vi "Execute_remote_call.vi"(0 "Traverse line":T3 {"Row Duration (mins)" format="%#.1f"; "Row No" min=0; "Trace Gas Concentration (%)" min=0.0 format="%#.2f"; "Emission Rate (l/min)" format="%#.2f"; "Tunnel Speed" format="%#.2f"; "Start X" format="%#.2f"; "Start Y" format="%#.2f"; "Start Z" format="%#.2f"; "End X" format="%#.2f"; "End Y" format="%#.2f"; "End Z" format="%#.2f"; "Averaging time (min)" min=0.0 format="%#.2f"}, 2 "Simulate/Run":T2, 3 "VI to run":path) -> (6 "Traverse Out":T3 {"Row Duration (mins)" format="%#.1f"; "Row No" min=0; "Trace Gas Concentration (%)" min=0.0 format="%#.2f"; "Emission Rate (l/min)" format="%#.2f"; "Tunnel Speed" format="%#.2f"; "Start X" format="%#.2f"; "Start Y" format="%#.2f"; "Start Z" format="%#.2f"; "End X" format="%#.2f"; "End Y" format="%#.2f"; "End Z" format="%#.2f"; "Averaging time (min)" min=0.0 format="%#.2f"}, 7 "Status":T1, 8 "Error Messages":string)   [LabVIEW 2012]
uses:
  Traverse_cluster.ctl
  Spacing.ctl
  Controls/Multi_run_mode.ctl
  Controls/User_Specific_mode.ctl
  Multi_Run_Status.ctl
panel:
  # "X           Y            Z"
  # "Start"
  # "End"
  # "X           Y            Z"
  # "Start"
  # "End"
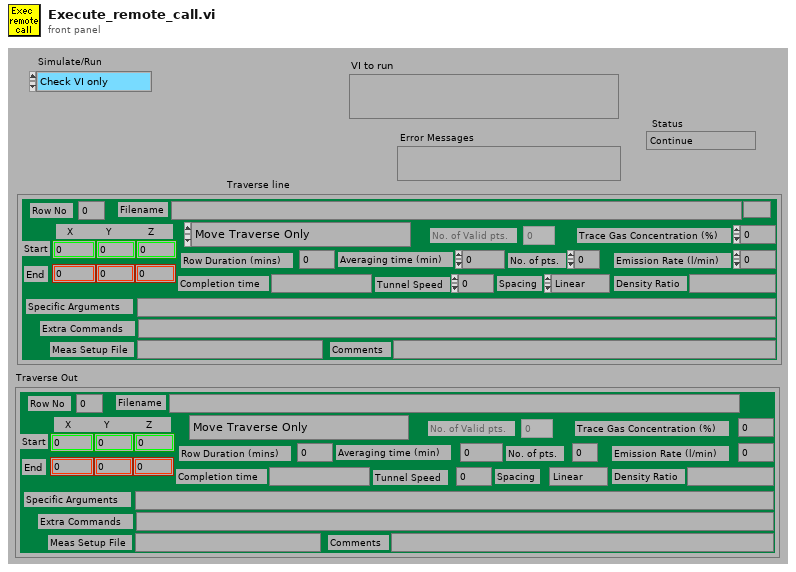
[diagram p1: front panel]
types:
  T1 = typedef "Multi_Run_Status.ctl" = enum16{"Continue", "Jump to Next Point", "Jump to Next Row", "Jump To Fall Back", "Terminate Run"}
  T2 = typedef "User_Specific_mode.ctl" = enum16{"Check VI only", "Run VI"}
  T3 = typedef "Traverse_cluster.ctl" = cluster{"Start X":dbl, "Start Y":dbl, "Start Z":dbl, "End X":dbl, "End Y":dbl, "End Z":dbl, "No. of pts.":i32, "Spacing":T4, "Filename":path, "Tunnel Speed":dbl, "Averaging time (min)":dbl, "Extra Commands":string, "Specific Arguments":string, "Emission Rate (l/min)":dbl, "Trace Gas Concentration (%)":dbl, "Density Ratio":string, "Comments":string, "Row No":i32, "Row Type Selector":T5, "Completion time":string, "Row Duration (mins)":dbl, "No. of Valid pts.":i32, "Meas Setup File":string}
  T4 = typedef "Spacing.ctl" = enum16{"Linear", "Log", "Gauss", "Specified", "N/A"}
  T5 = typedef "Multi_run_mode.ctl" = enum16{"Move Traverse Only", "Set Tunnel Speed Only", "Set Source Only", "Set Measurement Conditions", "Single Measurement", "Vertical Profile", "Lateral Profile", "Longitudinal Profile", "Explore Volume", "Multi-Axis Profile", "Auto Calibrate", "Meas Fast FID Bkgnd", "Check Beam Power", "Scanning Valve Measurement", "Run VI Named:", "Set ADAM Ch", "Wait (minutes)", "Send Message", "Synchronize With:", "Fall Back to this Row", "Turn Off Row Repeating", "Blank Row", "Traverse 3D Volume"}
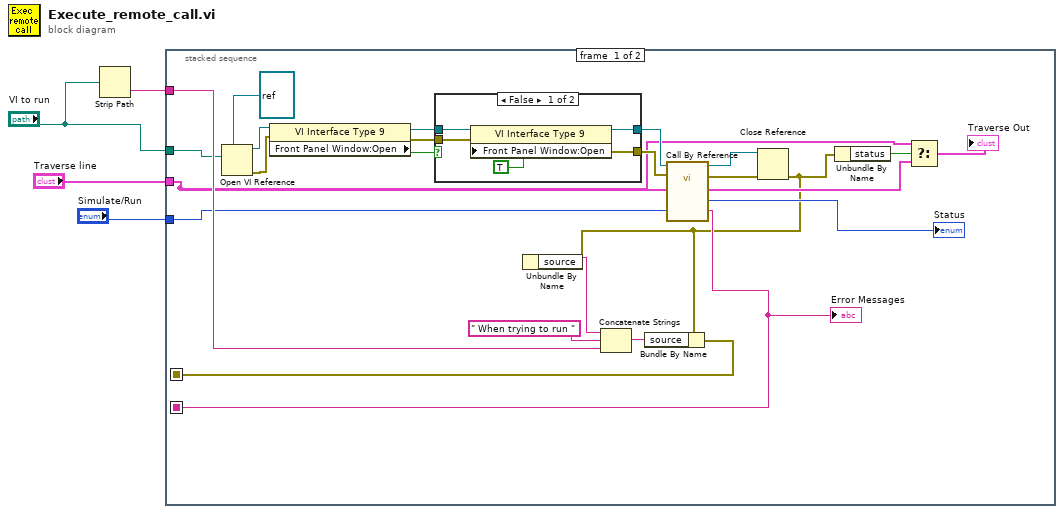
[diagram p0: block diagram]
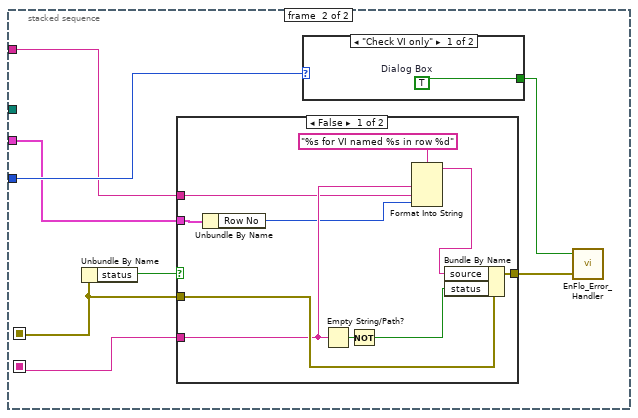
[diagram p3: hidden frame]
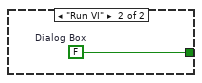
[diagram p4: hidden frame]
diagram:
  n1 = Strip Path(path="VI to run") -> (name=w2:string)  [unwired: 1 out]
  n2 = stacked-sequence {
    seq-local: [w20 _] -> [_ w38]
    seq-local: [w23 _] -> [_ w39]
    tunnel: w2 -> [w24 w37]
    tunnel: "Simulate/Run" -> [w22 w42]
    tunnel: "VI to run" -> [w21 _]
    tunnel: "Traverse line" -> [w6 w36]
    frame #0 {
      n3 = Open VI Reference(type specifier VI Refnum (for type only)=refnum<vi> refnum, vi path=w21) -> (vi reference=w8:refnum<vi>, error out=w10:errorcluster)  [unwired: 2 in, 2 out]
      n4 = property class="VI Interface Type 9"(reference=w8, error in=w10) -> (reference out=w12:refnum<vi>, error out=w13:errorcluster, "Front Panel Window:Open"=w11:bool)
      n5 = case shown="False" w11 {
        tunnel: w12 -> [w33 w35]
        tunnel: w13 -> [w32 w34]
        tunnel: [w31 w35] -> w7
        tunnel: [w29 w34] -> w9
        frame False {
          n6 = property class="VI Interface Type 9"(reference=w33, error in=w32, "Front Panel Window:Open"=TRUE) -> (reference out=w31:refnum<vi>, error out=w29:errorcluster)
        }
        frame True {
        }
      }
      n7 = call-by-ref "?"(reference=w7, error in=w9, "Simulate/Run"=w22, "Traverse line"=w6) -> (reference out=w25:refnum<vi>, error out=w15:errorcluster, "Error Messages"=w20:string, "Status"=→"Status":T1, "Traverse line Out"=w17:T3)  [unwired: 1 in]
      "Error Messages" <- w20
      n8 = Close Reference(reference=w25, error in (no error)=w15) -> (error out=w14:errorcluster)
      n9 = Unbundle By Name(w14) -> ("source"=w28:string)
      n10 = Concatenate Strings(w28, " When trying to run " ("Substring"), w24) -> (w26:string)
      n11 = Bundle By Name(cluster=w14, "source"=w26) -> (w23:errorcluster)
      n12 = Unbundle By Name(w14) -> ("status"=w18:bool)
      n13 = Select(t=w6, s=w18, f=w17) -> (s? t:f=→"Traverse Out":T3)
    }
    frame #1 {
      n14 = Unbundle By Name(w39) -> ("status"=w43:bool)
      n15 = case shown="False" w43 {
        tunnel: [w54 w56] -> w40
        tunnel: w39 -> [w55 w56]
        tunnel: w38 -> [w52 _]
        tunnel: w37 -> [w51 _]
        tunnel: w36 -> [w48 _]
        frame False {
          n16 = Unbundle By Name(w48) -> ("Row No"=w47:i32)
          n17 = Empty String/Path?(string/path=w52) -> (empty?=w53:bool)
          n18 = Not(x=w53) -> (.not. x?=w46:bool)
          n19 = Format Into String(format string="%s for VI named %s in row %d" ("Format String"), w52, w51, w47) -> (resulting string=w49:string)  [unwired: 2 in, 1 out]
          n20 = Bundle By Name(cluster=w55, "source"=w49, "status"=w46) -> (w54:errorcluster)
        }
        frame True {
        }
      }
      n21 = case shown="\"Check VI only\"" w42 {
        tunnel: [w44 w45] -> w41
        frame "Check VI only" {
          w44 = TRUE  # Dialog Box
        }
        frame "Run VI" {
          w45 = FALSE  # Dialog Box
        }
      }
      n22 = call "EnFlo_Error_Handler.vi"("error in (no error)"=w40, "Dialog Box (T)"=w41) -> ()  [unwired: 1 in, 3 out]
    }
  }
